vi "Unit Test.vi"() -> ()   [LabVIEW 2018]
uses:
  MSOX6004.lvclass
  PPLs/Oscilloscope/Parent/Oscilloscope.lvlibp/Custom Controls/Analog Channels.ctl
  PPLs/Oscilloscope/Parent/Oscilloscope.lvlibp/Custom Controls/Run Control.ctl
  PPLs/Oscilloscope/Parent/Oscilloscope.lvlibp/Custom Controls/Volts per Division.ctl
  PPLs/Oscilloscope/Parent/Oscilloscope.lvlibp/Custom Controls/Select Cursor.ctl
  PPLs/Oscilloscope/Parent/Oscilloscope.lvlibp/Custom Controls/Measurement.ctl
  PPLs/Oscilloscope/Parent/Oscilloscope.lvlibp/Custom Controls/Target Data.ctl
  PPLs/Oscilloscope/Parent/Oscilloscope.lvlibp/Oscilloscope.lvclass
  C:/Projects/LabVIEW/PPLs/Oscilloscope/Parent/Oscilloscope.lvlibp/Oscilloscope.lvclass
  PPLs/Oscilloscope/Parent/Oscilloscope.lvlibp
panel:
  out "Array":string[](array[string])
  out "loops":i32
  in  "loops":i32
  out "Jitter":dbl
  in  "No. Periods":u32
  in  "Target Data":T1
  in  "Measurement 2":T2
  out "Measurement":dbl
  out "Position":dbl format="%.9f"
  in  "Cursor":T3
  in  "Intensity (1-100)":i8=1 min=1 max=100 step=1
  in  "Label":string
  in  "Offset Divisions":dbl
  out "Status Array":bool[](array[boolean])
  in  "Trigger Level (0.0 V)":dbl=2.2 format="%#_13g"
  in  "Trigger Slope (0: Rising)":u16(ring) items=["Rising", "Falling", "Either"]
  in  "Secs/div":dbl
  in  "V/div":T4
  in  "Active Channel(s)":T5[](array[typedef])
  in  "stop":bool
  in  "Run Control":T6
  in  "Channel":T5
  out "Waveform Graph":waveform(dbl)[](graph)
  in  "Screen Shot Path":path
  in  "Lock Controls?":bool
  out "error out":errorcluster
  out "MSOX6004 out":refnum<class "MSOX6004.lvclass">
  in  "Resource":refnum<visa-resource-name>="TCPIP0::192.168.0.50::INSTR"
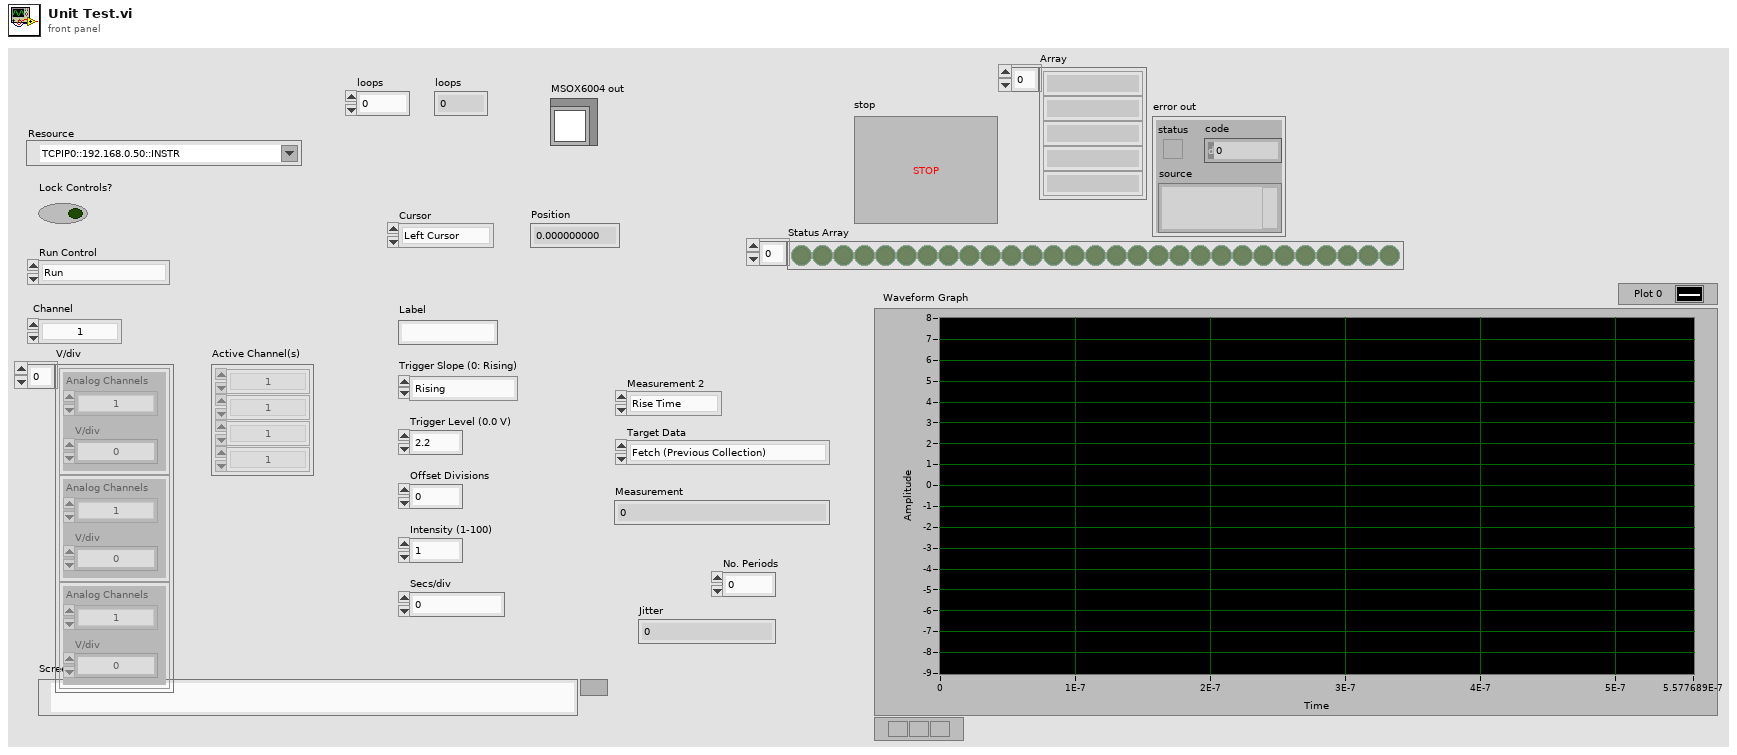
[diagram p1: front panel]
types:
  T1 = typedef "Oscilloscope.lvlibp/Target Data.ctl" = enum16{"Fetch (Previous Collection)", "Measure (New Collection)"}
  T2 = typedef "Oscilloscope.lvlibp/Measurement.ctl" = enum16{"Rise Time", "Fall Time", "Frequency", "Period", "RMS (V)", "Peak-Peak (V)", "Max (V)", "Min (V)", "High State (V)", "Low State (V)", "Average (V)", "Width (Negative)", "Width (Positive)", "Duty Cycle (Negative)", "Duty Cycle (Positive)", "Amplitude", "Cycle RMS (V)", "Cycle Avg (V)", "Overshoot", "Preshoot", "Time at Max", "Frequency Counter", "Time at Min", "Delay", "Value at Time", "Phase", "Time at Value", "Time of Edge", "Area", "Burst Width", "Falling Edge Count", "Rising Edge Count", "Falling Pulse Count", "Rising Pulse Count", "Std Dev", "Pulse Width"}
  T3 = typedef "Oscilloscope.lvlibp/Select Cursor.ctl" = enum16{"Left Cursor", "Right Cursor", "Top Cursor", "Bottom Cursor"}
  T4 = typedef "Oscilloscope.lvlibp/Volts per Division.ctl" = cluster{"Analog Channels":T5, "V/div":dbl}[]
  T5 = typedef "Oscilloscope.lvlibp/Analog Channels.ctl" = enum16{"1", "2", "3", "4", "5", "6", "7", "8", "9", "10", "11", "12", "13", "14", "15", "16"}
  T6 = typedef "Oscilloscope.lvlibp/Run Control.ctl" = enum16{"Run", "Single", "Stop"}
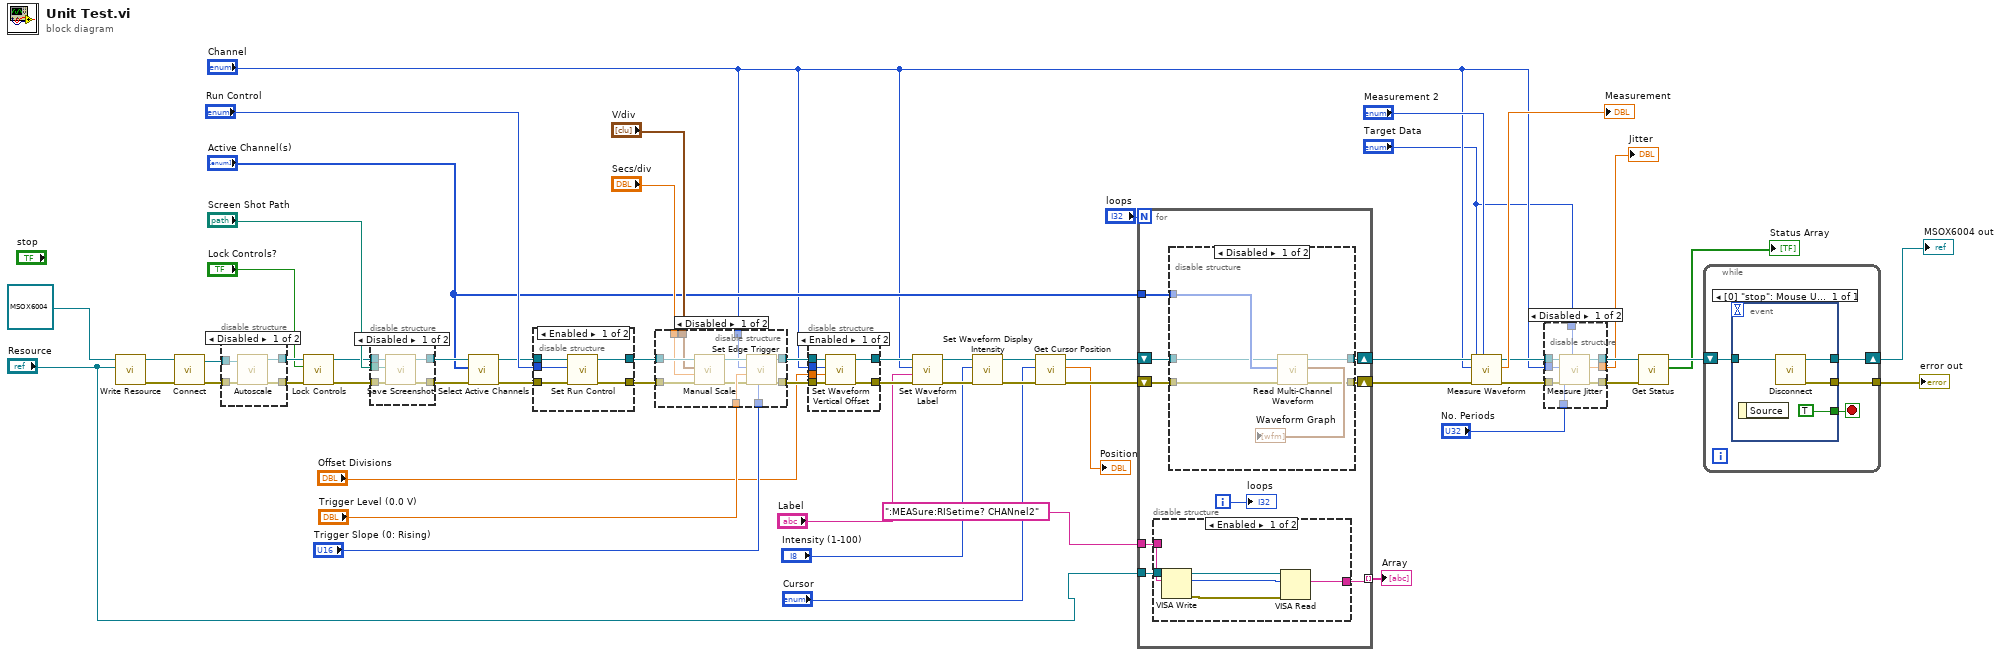
[diagram p0: block diagram]
diagram:
  n1 = call "Write Resource.vi"("Resource"="Resource", "Oscilloscope in"=refnum<class "MSOX6004.lvclass"> refnum ("MSOX6004.lvlib:MSOX6004.lvclass")) -> ("error out"=w56:errorcluster, "Oscilloscope out"=w57:refnum<class "MSOX6004.lvclass">)  [unwired: 8 in]
  n2 = call-dynamic "Connect.vi"("error in (no error)"=w56, "MSOX6004 in"=w57) -> ("error out"=w52:errorcluster, "MSOX6004 out"=w53:refnum<class "MSOX6004.lvclass">)  [unwired: 8 in]
  n3 = disable-structure shown="Disabled" {
    disable-tunnel: w53 -> [w62 w64]
    disable-tunnel: w52 -> [w61 w63]
    disable-tunnel: [w60 w64] -> w51
    disable-tunnel: [w59 w63] -> w50
    frame Disabled {
      n4 = call-dynamic "Autoscale.vi"("error in (no error)"=w61, "MSOX6004 in"=w62) -> ("error out"=w59:errorcluster, "MSOX6004 out"=w60:refnum<class "MSOX6004.lvclass">)  [unwired: 8 in]
    }
    frame Enabled {
    }
  }
  n5 = call-dynamic "Lock Controls.vi"("error in (no error)"=w50, "Lock Controls?"="Lock Controls?", "MSOX6004 in"=w51) -> ("error out"=w45:errorcluster, "MSOX6004 out"=w46:refnum<class "MSOX6004.lvclass">)  [unwired: 7 in]
  n6 = disable-structure shown="Disabled" {
    disable-tunnel: w46 -> [w69 w71]
    disable-tunnel: "Screen Shot Path" -> [w68 _]
    disable-tunnel: w45 -> [w67 w70]
    disable-tunnel: [w66 w71] -> w42
    disable-tunnel: [w65 w70] -> w44
    frame Disabled {
      n7 = call-dynamic "Save Screenshot.vi"("error in (no error)"=w67, "Screen Shot Path"=w68, "MSOX6004 in"=w69) -> ("error out"=w65:errorcluster, "MSOX6004 out"=w66:refnum<class "MSOX6004.lvclass">)  [unwired: 7 in]
    }
    frame Enabled {
    }
  }
  n8 = call-dynamic "Select Active Channels.vi"("error in (no error)"=w44, "Active Channel(s)"="Active Channel(s)", "MSOX6004 in"=w42) -> ("error out"=w43:errorcluster, "MSOX6004 out"=w41:refnum<class "MSOX6004.lvclass">)  [unwired: 7 in]
  n9 = disable-structure shown="Enabled" {
    disable-tunnel: [w76 w78] -> w40
    disable-tunnel: "Run Control" -> [w75 _]
    disable-tunnel: [w74 w77] -> w39
    disable-tunnel: w43 -> [w73 w77]
    disable-tunnel: w41 -> [w72 w78]
    frame Enabled {
      n10 = call-dynamic "Set Run Control.vi"("error in (no error)"=w73, "Run Control"=w75, "MSOX6004 in"=w72) -> ("error out"=w74:errorcluster, "MSOX6004 out"=w76:refnum<class "MSOX6004.lvclass">)  [unwired: 7 in]
    }
    frame Disabled {
    }
  }
  n11 = disable-structure shown="Disabled" {
    disable-tunnel: w40 -> [w89 w91]
    disable-tunnel: w39 -> [w88 w90]
    disable-tunnel: "V/div" -> [w87 _]
    disable-tunnel: "Secs/div" -> [w86 _]
    disable-tunnel: "Trigger Level (0.0 V)" -> [w84 _]
    disable-tunnel: "Trigger Slope (0: Rising)" -> [w83 _]
    disable-tunnel: [w81 w91] -> w31
    disable-tunnel: [w80 w90] -> w30
    disable-tunnel: "Channel" -> [w79 _]
    frame Disabled {
      n12 = call-dynamic "Manual Scale.vi"("error in (no error)"=w88, "Secs/div"=w86, "V/div"=w87, "MSOX6004 in"=w89) -> ("error out"=w82:errorcluster, "MSOX6004 out"=w85:refnum<class "MSOX6004.lvclass">)  [unwired: 6 in]
      n13 = call-dynamic "Set Edge Trigger.vi"("Trigger Slope (0: Rising)"=w83, "error in (no error)"=w82, "Trigger Level (0.0 V)"=w84, "Analog Channel"=w79, "MSOX6004 in"=w85) -> ("error out"=w80:errorcluster, "MSOX6004 out"=w81:refnum<class "MSOX6004.lvclass">)  [unwired: 5 in]
    }
    frame Enabled {
    }
  }
  n14 = disable-structure shown="Enabled" {
    disable-tunnel: w31 -> [w97 w99]
    disable-tunnel: [w96 w99] -> w28
    disable-tunnel: w30 -> [w95 w98]
    disable-tunnel: [w94 w98] -> w27
    disable-tunnel: "Channel" -> [w93 _]
    disable-tunnel: "Offset Divisions" -> [w92 _]
    frame Enabled {
      n15 = call-dynamic "Set Waveform Vertical Offset.vi"("error in (no error)"=w95, "Offset Divisions"=w92, "Analog Channels"=w93, "MSOX6004 in"=w97) -> ("error out"=w94:errorcluster, "MSOX6004 out"=w96:refnum<class "MSOX6004.lvclass">)  [unwired: 6 in]
    }
    frame Disabled {
    }
  }
  n16 = call-dynamic "Set Waveform Label.vi"("error in (no error)"=w27, "Label"="Label", "Analog Channels"="Channel", "MSOX6004 in"=w28) -> ("error out"=w24:errorcluster, "MSOX6004 out"=w25:refnum<class "MSOX6004.lvclass">)  [unwired: 6 in]
  n17 = call-dynamic "Set Waveform Display Intensity.vi"("error in (no error)"=w24, "Intensity (1-100)"="Intensity (1-100)", "MSOX6004 in"=w25) -> ("error out"=w21:errorcluster, "MSOX6004 out"=w22:refnum<class "MSOX6004.lvclass">)  [unwired: 7 in]
  n18 = call-dynamic "Get Cursor Position.vi"("error in (no error)"=w21, "Cursor"="Cursor", "MSOX6004 in"=w22) -> ("error out"=w19:errorcluster, "Position"=→"Position":dbl, "MSOX6004 out"=w20:refnum<class "MSOX6004.lvclass">)  [unwired: 6 in]
  n19 = for {
    N: "loops" -> [_]
    tunnel: "Active Channel(s)" -> [w108]
    shift-right: [w105] -> w16
    shift-left: w20 -> [w107]
    shift-right: [w104] -> w15
    shift-left: w19 -> [w106]
    tunnel: "Resource" -> [w102]
    tunnel: ":MEASure:RISetime? CHANnel2" ("write buffer") -> [w101]
    tunnel: [w100] -> w1 mode=indexing
    i -> [w103]
    n20 = disable-structure shown="Enabled" {
      disable-tunnel: w102 -> [w114 _]
      disable-tunnel: w101 -> [w113 _]
      disable-tunnel: [w110 _] -> w100
      frame Enabled {
        n21 = VISA Write(VISA resource name=w114, write buffer=w113) -> (VISA resource name out=w112:refnum<visa-resource-name>, return count=w109:u32, error out=w111:errorcluster)  [unwired: 1 in]
        n22 = VISA Read(VISA resource name=w112, byte count=w109, error in (no error)=w111) -> (read buffer=w110:string)  [unwired: 3 out]
      }
      frame Disabled {
      }
    }
    n23 = disable-structure shown="Disabled" {
      disable-tunnel: w108 -> [w120 _]
      disable-tunnel: w107 -> [w118 w122]
      disable-tunnel: w106 -> [w117 w121]
      disable-tunnel: [w116 w122] -> w105
      disable-tunnel: [w115 w121] -> w104
      frame Disabled {
        n24 = call-dynamic "Read Multi-Channel Waveform.vi"("error in (no error)"=w117, "Channels"=w120, "MSOX6004 in"=w118) -> ("error out"=w115:errorcluster, "Waveform"=→"Waveform Graph":waveform(dbl)[], "MSOX6004 out"=w116:refnum<class "MSOX6004.lvclass">)  [unwired: 6 in]
      }
      frame Enabled {
      }
    }
    "loops" <- w103
  }
  "Array" <- w1
  n25 = call-dynamic "Measure Waveform.vi"("Target Data"="Target Data", "error in (no error)"=w15, "Measurement"="Measurement 2", "Channel"="Channel", "MSOX6004 in"=w16) -> ("error out"=w10:errorcluster, "Measurement"=→"Measurement":dbl, "MSOX6004 out"=w12:refnum<class "MSOX6004.lvclass">)  [unwired: 4 in]
  n26 = disable-structure shown="Disabled" {
    disable-tunnel: w12 -> [w130 w132]
    disable-tunnel: [w129 w132] -> w11
    disable-tunnel: w10 -> [w128 w131]
    disable-tunnel: [w127 w131] -> w9
    disable-tunnel: "Channel" -> [w126 _]
    disable-tunnel: "No. Periods" -> [w125 _]
    disable-tunnel: "Target Data" -> [w124 _]
    disable-tunnel: [w123 _] -> w5
    frame Disabled {
      n27 = call-dynamic "Measure Jitter.vi"("Target Data"=w124, "error in (no error)"=w128, "No. Periods"=w125, "Channel"=w126, "MSOX6004 in"=w130) -> ("error out"=w127:errorcluster, "Jitter"=w123:dbl, "MSOX6004 out"=w129:refnum<class "MSOX6004.lvclass">)  [unwired: 4 in]
    }
    frame Enabled {
    }
  }
  "Jitter" <- w5
  n28 = call-dynamic "Get Status.vi"("error in (no error)"=w9, "MSOX6004 in"=w11) -> ("Status Array"=→"Status Array":bool[], "MSOX6004 out"=w33:refnum<class "MSOX6004.lvclass">)  [unwired: 7 in, 1 out]
  n29 = while {
    tunnel: [w135] -> w54
    shift-right: [w136] -> w55
    shift-left: w33 -> [w134]
    stop <- w133 stop-if-true
    n30 = event shown="[0] \"stop\": Mouse Up" {
      selector: _ -> [_]
      dyn-events: _ -> [_]
      timeout: _ -> [_]
      tunnel: [w140] -> w136
      tunnel: [w139] -> w135
      tunnel: w134 -> [w138]
      tunnel: [TRUE] -> w133
      event "stop": Mouse Up {
        n31 = event-data() -> ()  [unwired: 1 in, 1 out]
        n32 = call-dynamic "Disconnect.vi"("MSOX6004 in"=w138) -> ("error out"=w139:errorcluster, "MSOX6004 out"=w140:refnum<class "MSOX6004.lvclass">)  [unwired: 9 in]
      }
    }
  }
  "MSOX6004 out" <- w55
  "error out" <- w54
